vi "MSGR Global Send.vi"(0 "Msg":string, 5 "Parameters":string, 7 "Reply?":bool, 9 "ReplyQ":string, 11 "error in (no error)":errorcluster, 12 "timeout in ms (-1)":i32=-1) -> (8 "timed out?":bool, 15 "error out":errorcluster)   [LabVIEW 2018]
doc: "$Author::Richard Jennings $\n$Rev:: $\n$Date:: May, 2008 $\n\nOVERVIEW:\nReentrant VI to receive messages via a MSGR Q. If the Q does not exist this VI will create it, then wait for data.\n\nINPUTS (Controls):\n<name> - <short description of each control wired to connector pane>\n\nOUTPUTS (Indicators):\n<name> - <short description of each indicator wired to connector pane>\n\nCopyright 2008 - 2017 Jennings Embedded Servies. All rights reserved.\nAuthor makes no warranties or guarantees related to performance of the software.\nUSE AT YOUR OWN RISK\nwww.jembedded.com"
uses:
  MSGR Registry Control TypeDef.ctl
  MSGR Q Data TypeDef.ctl
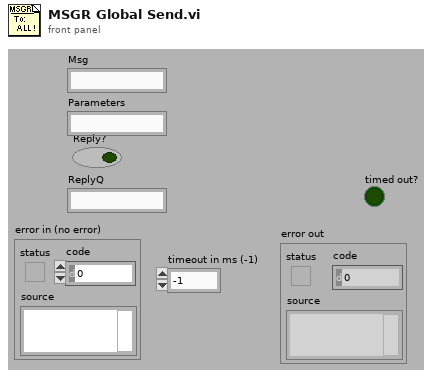
[diagram p1: front panel]
types:
  T1 = typedef "MSGR Registry Control TypeDef.ctl" = enum16{"reset", "register", "get data", "set data", "unregister", "test", "get objects"}
  T2 = typedef "MSGR Q Data TypeDef.ctl" = cluster{"Msg":string, "Parameters":string, "Reply?":bool, "ReplyQ":string}
  T3 = typedef "MSGR Q Name TypeDef.ctl" = string
  T4 = typedef "MSGR Q Ref TypeDef.ctl" = refnum<queue>
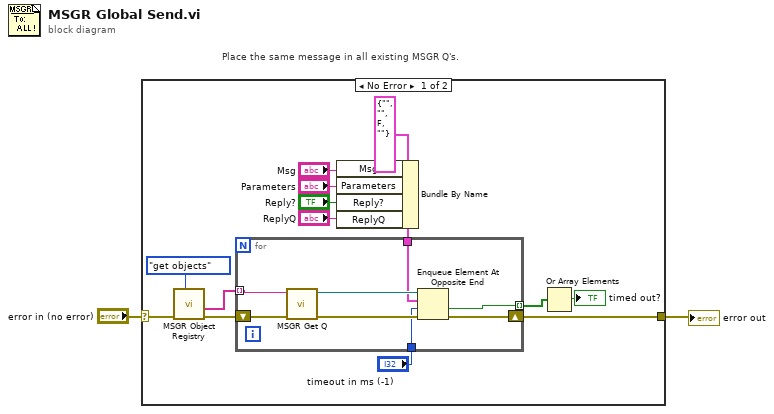
[diagram p0: block diagram]
diagram:
  # "Place the same message in all existing MSGR Q's."
  n1 = case shown="No Error" "error in (no error)" {
    selector: "error in (no error)" -> [w16 w25]
    tunnel: [w10 w25] -> w2
    frame No Error {
      n2 = call "MSGR Object Registry.vi"("function (get data)"=MSGR_Registry_Control_TypeDef."get objects", "error in (no error)"=w16) -> ("error out"=w9:errorcluster, "MSGR Q names"=w7:T3[])  [unwired: 2 in, 6 out]
      n3 = Bundle By Name(cluster=T2 {"Msg"="", "Parameters"="", "Reply?"=FALSE, "ReplyQ"=""} ("element"), "Msg"="Msg", "Parameters"="Parameters", "Reply?"="Reply?", "ReplyQ"="ReplyQ") -> (w14:T2)
      n4 = for {
        tunnel: w14 -> [w21]
        shift-right: [w20] -> w10
        shift-left: w9 -> [w24]
        tunnel: w7 -> [w19] mode=indexing
        tunnel: [w18] -> w6 mode=indexing
        tunnel: "timeout in ms (-1)" -> [w17]
        n5 = call "MSGR Get Q.vi"("error in (no error)"=w24, "MSGR Q name"=w19) -> ("error out"=w23:errorcluster, "MSGR Q"=w22:T4)  [unwired: 8 out]
        n6 = Enqueue Element At Opposite End(queue=w22, element=w21, timeout in ms (-1)=w17, error in (no error)=w23) -> (timed out?=w18:bool, error out=w20:errorcluster)  [unwired: 1 out]
      }
      n7 = Or Array Elements(Boolean array=w6) -> (logical OR=→"timed out?":bool)
    }
    frame Error {
    }
  }
  "error out" <- w2
